vi "Perform Work.vi"(8 "error in (no error)":errorcluster, 9 "Initialize":bool, 10 "Reply to":refnum<class "Result Reply Msg.lvclass">, 11 "Instrument Recorder in":refnum<class "Instrument Actor.lvclass">) -> (0 "error out":errorcluster, 3 "Instrument Recorder out":refnum<class "Instrument Actor.lvclass">)   [LabVIEW 2016, in "Instrument Actor.lvclass"]
uses:
  Instrument Actor.lvclass
  Template Module Messages/Result Reply Msg/Result Reply Msg.lvclass
  Worker/Worker.lvclass
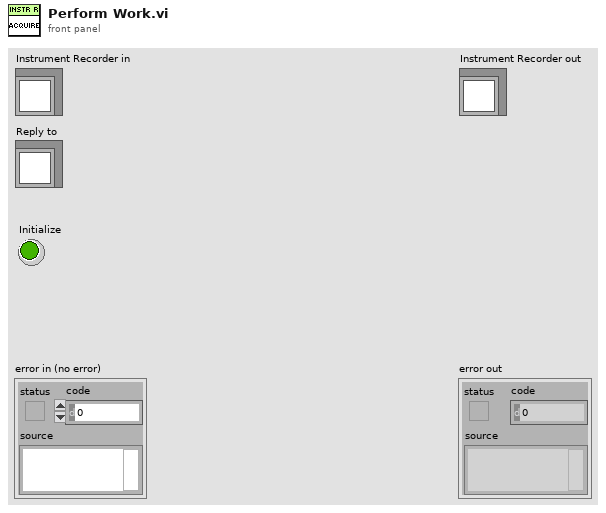
[diagram p1: front panel]
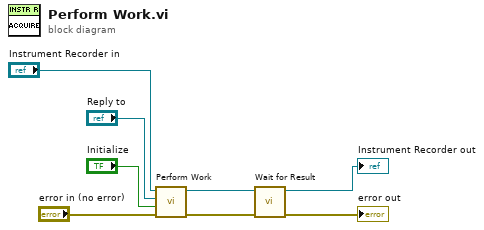
[diagram p0: block diagram]
diagram:
  n1 = call-parent "Perform Work.vi"("error in (no error)"="error in (no error)", "Initialize"="Initialize", "Reply to"="Reply to", "Measure Object in"="Instrument Recorder in") -> ("error out"=w4:errorcluster, "Measure Object out"=w3:refnum<class "Instrument Actor.lvclass">)  [unwired: 6 in]
  n2 = call-dynamic "Wait for Result.vi"("error in (no error)"=w4, "Instrument Recorder in"=w3) -> ("error out"=→"error out":errorcluster, "Instrument Recorder out"=→"Instrument Recorder out":refnum<class "Instrument Actor.lvclass">)  [unwired: 8 in]
